vi "can test.vi"() -> ()   [LabVIEW 2019]
uses:
  Type Defs/CAN Mode.ctl
panel:
  out "appended array 2":u32[](array[numeric]) format="%.0x"
  out "appended array":u8[][](array[numeric]) format="%.0x"
  out "error out":errorcluster
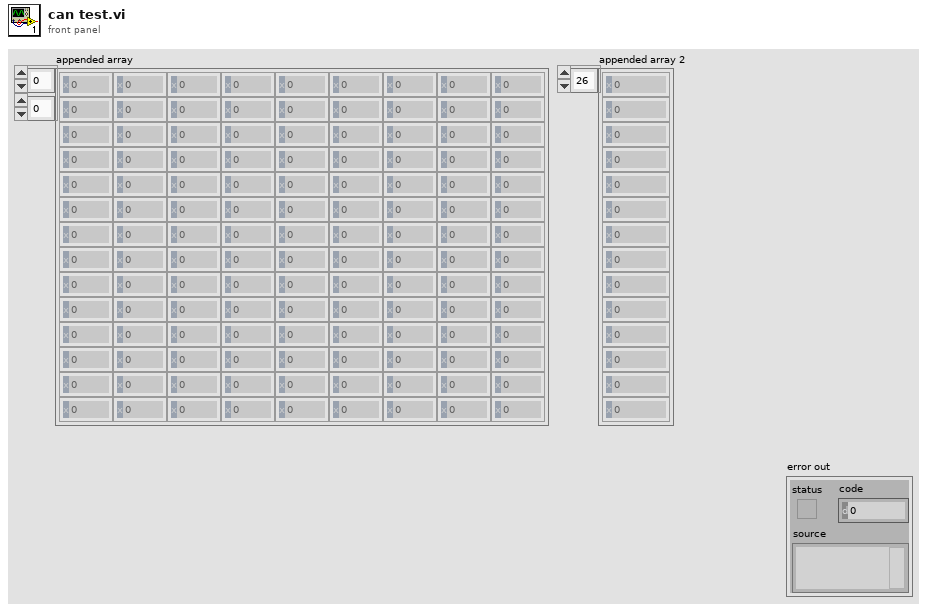
[diagram p1: front panel]
types:
  T1 = typedef "CAN Mode.ctl" = enum16{"Init", "Read", "Write", "Close"}
  T2 = typedef "CANFrameControl.ctl" = cluster{"identifier":u32, "extended?":bool, "type":u8, "payload":u8[]}
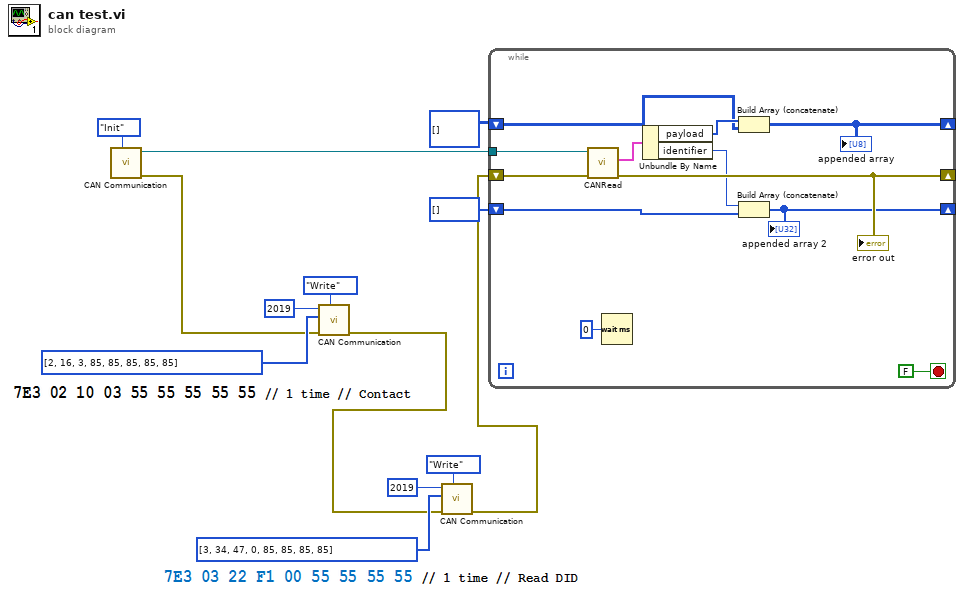
[diagram p0: block diagram]
diagram:
  n1 = call "CAN Communication.vi"("CAN Mode"=CAN_Mode."Init") -> ("Error OUT"=w7:errorcluster, "CAN Ref"=w6:refnum<k20>)  [unwired: 9 in]
  n2 = call "CAN Communication.vi"("CAN Mode"=CAN_Mode."Write", "Error IN"=w7, "Message"=u8[] [2, 16, 3, 85, 85, 85, 85, 85] ("array"), "Arbitration ID"=u32 2019 ("CAN Addres to Xmit\nSpeed CMD (Hex) 2")) -> ("Error OUT"=w2:errorcluster)  [unwired: 6 in, 1 out]
  n3 = call "CAN Communication.vi"("CAN Mode"=CAN_Mode."Write", "Error IN"=w2, "Message"=u8[] [3, 34, 47, 0, 85, 85, 85, 85] ("array"), "Arbitration ID"=u32 2019 ("CAN Addres to Xmit\nSpeed CMD (Hex) 2")) -> ("Error OUT"=w1:errorcluster)  [unwired: 6 in, 1 out]
  n4 = while {
    tunnel: w6 -> [w24]
    shift-right: [w22] -> _
    shift-left: w1 -> [w23]
    shift-right: [w19] -> _
    shift-left: u8[][] [] -> [w17]
    shift-right: [w15] -> _
    shift-left: u32[] [] -> [w14]
    stop <- FALSE stop-if-true
    n5 = call <vilib>:"CANRead.vi"("error in (no error)"=w23, "interface object in"=w24) -> ("error out"=w22:errorcluster, "CAN frame"=w20:T2)  [unwired: 6 in, 2 out]
    "error out" <- w22
    n6 = Wait (ms)(milliseconds to wait=u32 0) -> ()  [unwired: 1 out]
    n7 = Unbundle By Name(w20) -> ("payload"=w18:u8[], "identifier"=w16:u32)
    n8 = Build Array (concatenate)(w18, w17) -> (w19:u8[][])
    "appended array" <- w19
    n9 = Build Array (concatenate)(w16, w14) -> (w15:u32[])
    "appended array 2" <- w15
  }
